vi "PWM_Manual.vi"() -> ()   [LabVIEW 2014]
uses:
  <vilib>/LabVIEW Interface for Arduino/Type Defs/Pin Mode.ctl
  <vilib>/LabVIEW Interface for Arduino/LabVIEW Interface for Arduino.lvlib
panel:
  in  "VISA resource":refnum<visa-resource-name>
  in  "Slide":dbl(slide) scale=0.0..20.0
  out "Waveform Chart":dynamicdata(graph)
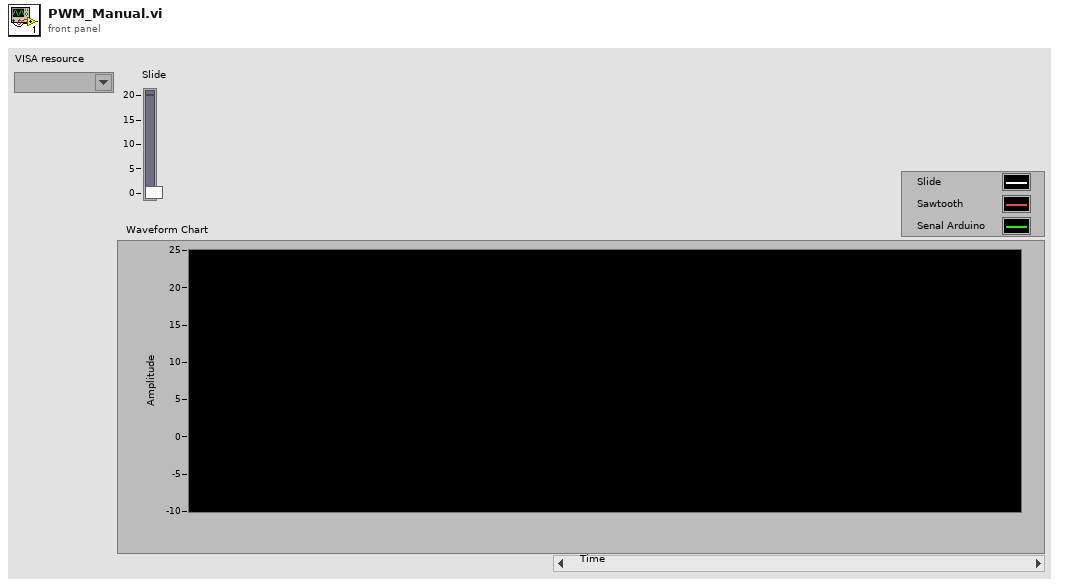
[diagram p1: front panel]
types:
  T1 = typedef "LabVIEW Interface for Arduino.lvlib/Pin Mode.ctl" = enum8{"Input", "Output"}
  T2 = typedef "LabVIEW Interface for Arduino.lvlib/Arduino Resource.ctl" = cluster{"VISA resource":refnum<visa-resource-name>, "Board Type":T3, "Connection Type":enum8{"USB / Serial"}, "Bytes Per Packet (15)":u8}
  T3 = typedef "LabVIEW Interface for Arduino.lvlib/Board Type.ctl" = enum16{"Uno", "Dimuelanove w/Atmega 328", "Mega 2560"}
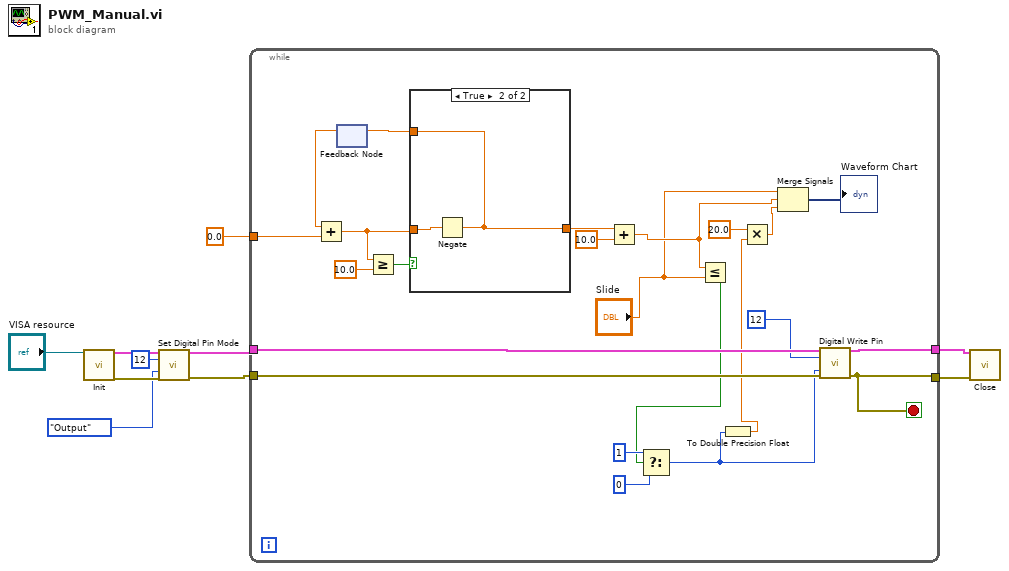
[diagram p0: block diagram]
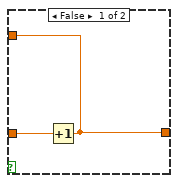
[diagram p2: hidden frame]
diagram:
  n1 = call <vilib>:"Init.vi"("VISA resource"="VISA resource") -> ("Arduino Resource"=w6:T2, "error out"=w5:errorcluster)  [unwired: 17 in]
  n2 = call <vilib>:"Set Digital Pin Mode.vi"("Arduino Resource"=w6, "Digital I/O Pin"=u8 12, "Pin Mode (Input)"=Pin_Mode."Output", "error in"=w5) -> ("Arduino Resource"=w3:T2, "error out"=w4:errorcluster)  [unwired: 10 in]
  n3 = while {
    tunnel: 0.0 -> [w33]
    tunnel: w4 -> [w27]
    tunnel: w3 -> [w25]
    tunnel: [w26] -> w9
    tunnel: [w24] -> w8
    stop <- w26 stop-if-true
    n4 = feedback #1() -> (w32:dbl)  [unwired: 1 in]
    n5 = Add(x=w32, y=w33) -> (x+y=w28:dbl)
    n6 = Greater Or Equal?(x=w28, y=10.0) -> (x >= y?=w31:bool)
    n7 = case shown="True" w31 {
      tunnel: w28 -> [w35 w37]
      tunnel: [w34 w36] -> w29
      tunnel: [w34 w36] -> w19
      frame False {
        n8 = Increment(x=w35) -> (x+1=w34:dbl)
      }
      frame True {
        n9 = Negate(x=w37) -> (-x=w36:dbl)
      }
    }
    n10 = feedback-in #1(w29) -> ()
    n11 = Add(x=w19, y=10.0) -> (x+y=w16:dbl)
    n12 = Less Or Equal?(x=w16, y="Slide") -> (x <= y?=w20:bool)
    n13 = Select(t=u8 1, s=w20, f=u8 0) -> (s? t:f=w12:u8)
    n14 = To Double Precision Float(number=w12) -> (double precision float=w11:dbl)
    n15 = Multiply(x=20.0, y=w11) -> (x*y=w14:dbl)
    n16 = Merge Signals("Slide", w16, w14) -> (→"Waveform Chart":dynamicdata)
    n17 = call <vilib>:"Digital Write Pin.vi"("Arduino Resource"=w25, "Digital I/O Pin (0)"=u8 12, "Value (0)"=w12, "error in"=w27) -> ("Arduino Resource"=w24:T2, "error out"=w26:errorcluster)  [unwired: 10 in]
  }
  n18 = call <vilib>:"Close.vi"("Arduino Resource"=w8, "error in"=w9) -> ()  [unwired: 13 in, 1 out]
